vi "transform string to byte array.vi"() -> ()   [LabVIEW 2021]
panel:
  out "data 3":u8[](array[numeric])
  out "t1 3":u32
  out "data 2":u8[](array[numeric])
  out "t1 2":u32
  out "data":u8[](array[numeric])
  out "t1":u32
  in  "Numeric":i32=100000
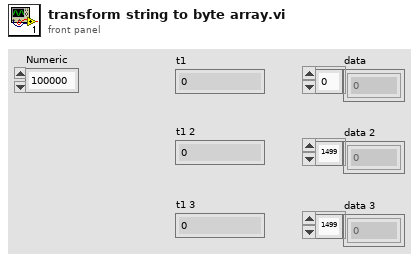
[diagram p1: front panel]
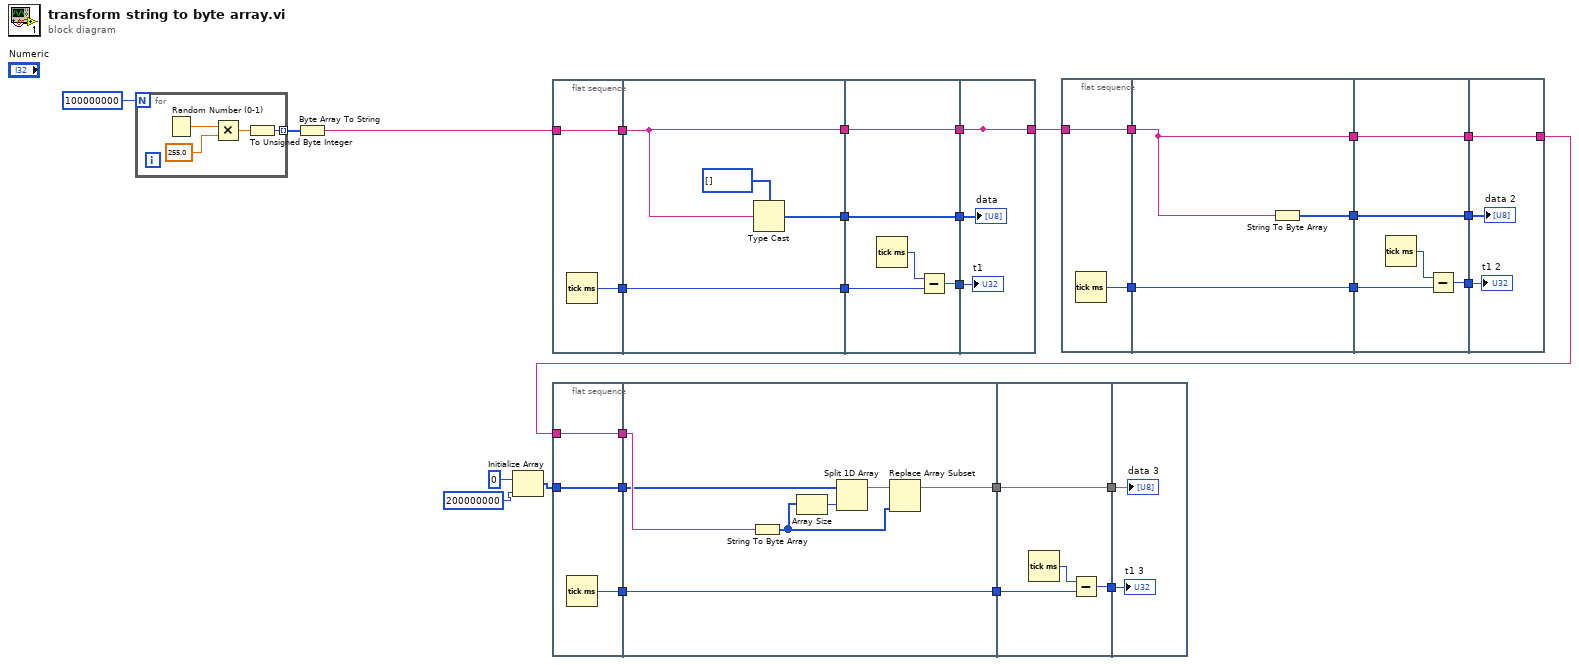
[diagram p0: block diagram]
diagram:
  n1 = for {
    N: 100000000 -> [_]
    tunnel: [w32] -> w2 mode=indexing
    n2 = Random Number (0-1)() -> (number: 0 to 1=w35:dbl)
    n3 = Multiply(x=w35, y=255.0) -> (x*y=w33:dbl)
    n4 = To Unsigned Byte Integer(number=w33) -> (unsigned 8bit integer=w32:u8)
  }
  n5 = Byte Array To String(unsigned byte array=w2) -> (string=w31:string)
  n6 = Initialize Array(u8 0 ("element"), 200000000 ("dimension size")) -> (w5:u8[])
  n7 = flat-sequence {
    tunnel: w31 -> [w37]
    tunnel: [w37] -> w30
    tunnel: [w36] -> w29
    tunnel: w30 -> [w39]
    tunnel: w29 -> [w41]
    tunnel: [w41] -> w28
    tunnel: [w40] -> w27
    tunnel: [w39] -> w17
    tunnel: w28 -> [w43]
    tunnel: w27 -> [w45]
    tunnel: [w46] -> w26
    tunnel: [w45] -> w25
    tunnel: [w42] -> w18
    tunnel: w17 -> [w42]
    tunnel: w26 -> [w48]
    tunnel: w25 -> [w49]
    tunnel: [w47] -> _
    tunnel: w18 -> [w47]
    tunnel: [w47] -> w16
    frame #0 {
      n8 = Tick Count (ms)() -> (millisecond timer value=w36:u32)
    }
    frame #1 {
      n9 = Type Cast(type=u8[] [] ("data"), x=w39) -> (*(type *) &x=w40:u8[])
    }
    frame #2 {
      n10 = Tick Count (ms)() -> (millisecond timer value=w44:u32)
      n11 = Subtract(x=w44, y=w43) -> (x-y=w46:u32)
    }
    frame #3 {
      "data" <- w49
      "t1" <- w48
    }
  }
  n12 = flat-sequence {
    tunnel: w7 -> [w52]
    tunnel: [w52] -> w13
    tunnel: [w51] -> w12
    tunnel: [w50] -> w6
    tunnel: w5 -> [w50]
    tunnel: w13 -> [w58]
    tunnel: w12 -> [w59]
    tunnel: [w59] -> w11
    tunnel: [w56] -> w10
    tunnel: w6 -> [w57]
    tunnel: w11 -> [w60]
    tunnel: w10 -> [w62]
    tunnel: [w63] -> w9
    tunnel: [w62] -> w8
    tunnel: w9 -> [w64]
    tunnel: w8 -> [w65]
    frame #0 {
      n13 = Tick Count (ms)() -> (millisecond timer value=w51:u32)
    }
    frame #1 {
      n14 = String To Byte Array(string=w58) -> (unsigned byte array=w55:u8[])
      n15 = Array Size(array=w55) -> (size(s)=w54:i32)
      n16 = Split 1D Array(array=w57, index=w54) -> (first subarray=w53:u8[])  [unwired: 1 out]
      n17 = Replace Array Subset(array=w53, new element=w55) -> (w56:u8[])  [unwired: 1 in]
    }
    frame #2 {
      n18 = Tick Count (ms)() -> (millisecond timer value=w61:u32)
      n19 = Subtract(x=w61, y=w60) -> (x-y=w63:u32)
    }
    frame #3 {
      "data 3" <- w65
      "t1 3" <- w64
    }
  }
  n20 = flat-sequence {
    tunnel: w16 -> [w67]
    tunnel: [w67] -> w24
    tunnel: [w66] -> w23
    tunnel: w24 -> [w68]
    tunnel: w23 -> [w70]
    tunnel: [w70] -> w22
    tunnel: [w69] -> w21
    tunnel: [w68] -> w14
    tunnel: w22 -> [w72]
    tunnel: w21 -> [w74]
    tunnel: [w75] -> w20
    tunnel: [w74] -> w19
    tunnel: [w71] -> w15
    tunnel: w14 -> [w71]
    tunnel: w20 -> [w77]
    tunnel: w19 -> [w78]
    tunnel: [w76] -> w7
    tunnel: w15 -> [w76]
    frame #0 {
      n21 = Tick Count (ms)() -> (millisecond timer value=w66:u32)
    }
    frame #1 {
      n22 = String To Byte Array(string=w68) -> (unsigned byte array=w69:u8[])
    }
    frame #2 {
      n23 = Tick Count (ms)() -> (millisecond timer value=w73:u32)
      n24 = Subtract(x=w73, y=w72) -> (x-y=w75:u32)
    }
    frame #3 {
      "data 2" <- w78
      "t1 2" <- w77
    }
  }
